vi "elimina riga da tabella.vi"(9 "indice riga":i32, 10 "tab":string, 11 "Res freddo res meter in":string[][](array[string])) -> (2 "riga eliminata":string[](array[string]), 3 "Array":string[][](array[string]))   [LabVIEW 2019]
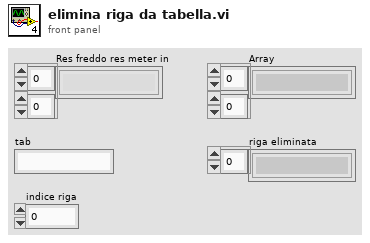
[diagram p1: front panel]
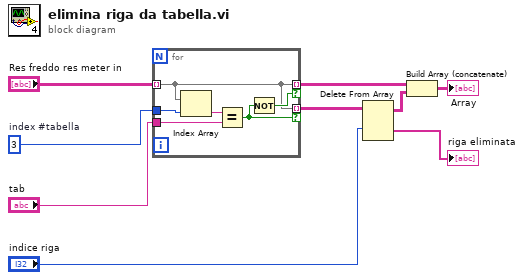
[diagram p0: block diagram]
diagram:
  w9 = 3  # index #tabella
  n1 = for {
    tunnel: "Res freddo res meter in" -> [w12] mode=indexing
    tunnel: [w12] -> w5 mode=indexing if=w13
    tunnel: "tab" -> [w14]
    tunnel: [w12] -> w3 mode=indexing if=w11
    tunnel: w9 -> [w10]
    n2 = Index Array(array=w12, index=w10) -> (element=w15:string)
    n3 = Equal?(x=w15, y=w14) -> (x = y?=w11:bool)
    n4 = Not(x=w11) -> (.not. x?=w13:bool)
  }
  n5 = Delete From Array(array=w3, index (row)="indice riga") -> (deleted portion=→"riga eliminata":string[], array with subset deleted=w6:string[][])  [unwired: 2 in]
  n6 = Build Array (concatenate)(w5, w6) -> (→"Array":string[][])
